vi "SetLimits.vi"(8 "error in (no error)":errorcluster, 10 "Limits":cluster{"Upper limit":dbl, "Lower limit":dbl}[](array[cluster]), 11 "Stage in":refnum<class "Stage.lvclass">) -> (0 "error out":errorcluster, 3 "Stage out":refnum<class "Stage.lvclass">)   [LabVIEW 2020, in "Stage.lvlib" / "Stage.lvclass"]
uses:
  Stage.lvclass
  Stage.lvclass/Stage.ctl
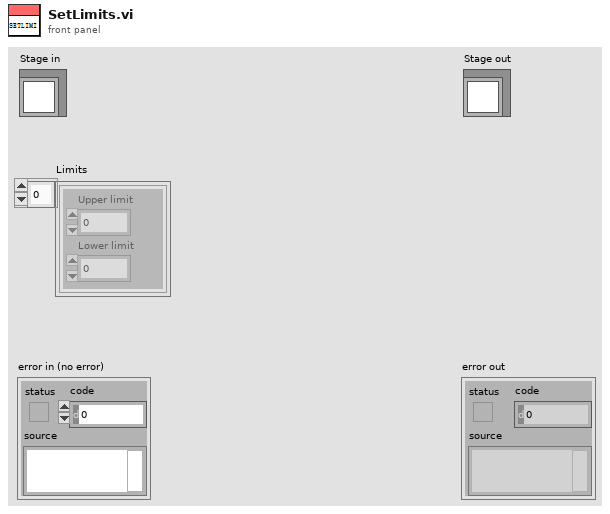
[diagram p1: front panel]
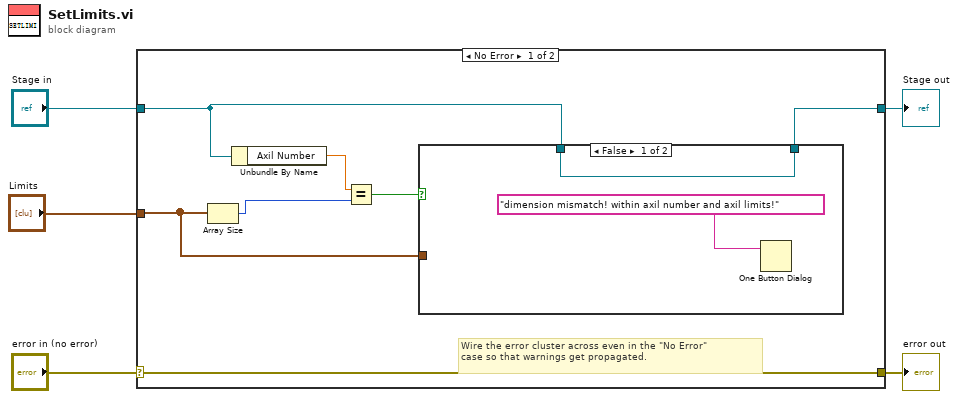
[diagram p0: block diagram]
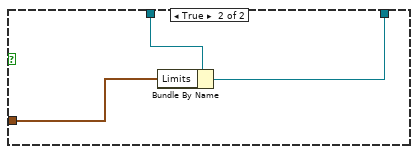
[diagram p2: hidden frame]
diagram:
  n1 = case shown="No Error" "error in (no error)" {
    selector: "error in (no error)" -> [w12 w19]
    tunnel: [w12 w19] -> w4
    tunnel: [w8 w18] -> w2
    tunnel: "Stage in" -> [w7 w18]
    tunnel: "Limits" -> [w6 _]
    frame No Error {
      # "Wire the error cluster across even in the \"No Error\"\ncase so that warnings get propagated."
      n2 = Array Size(array=w6) -> (size(s)=w10:i32)
      n3 = Unbundle By Name(w7) -> ("Axil Number"=w11:dbl)
      n4 = Equal?(x=w11, y=w10) -> (x = y?=w9:bool)
      n5 = case shown="False" w9 {
        tunnel: w7 -> [w13 w17]
        tunnel: [w13 w16] -> w8
        tunnel: w6 -> [_ w15]
        frame False {
          n6 = One Button Dialog(message="dimension mismatch! within axil number and axil limits!") -> ()  [unwired: 1 in, 1 out]
        }
        frame True {
          n7 = Bundle By Name(cluster=w17, "Limits"=w15) -> (w16:refnum<class "Stage.lvclass">)
        }
      }
    }
    frame Error {
    }
  }
  "error out" <- w4
  "Stage out" <- w2
